vi "Begin.vi"(8 "error in (no error)":errorcluster, 11 "Grabber in":refnum<class "Grabber.lvclass">) -> (0 "error out":errorcluster, 3 "Grabber out":refnum<class "Grabber.lvclass">)   [LabVIEW 2013, in "Grabber.lvclass"]
uses:
  Grabber.lvclass
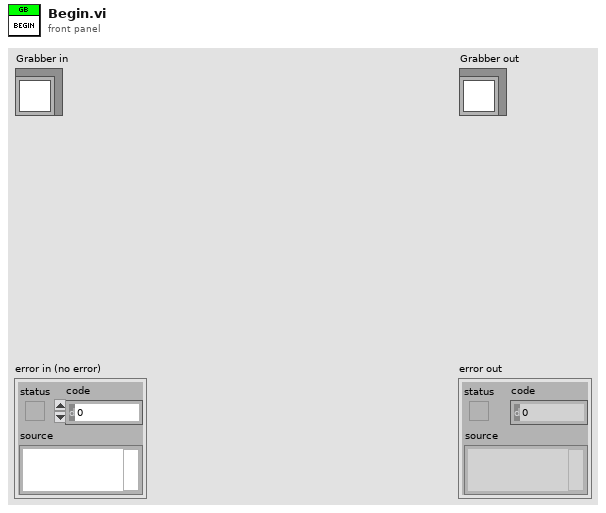
[diagram p1: front panel]
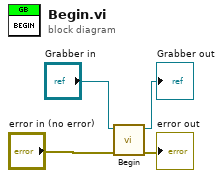
[diagram p0: block diagram]
diagram:
  n1 = call-dynamic "Begin.vi"("error in (no error)"="error in (no error)", "Grabber in"="Grabber in") -> ("error out"=→"error out":errorcluster, "Grabber out"=→"Grabber out":refnum<class "Grabber.lvclass">)  [unwired: 8 in]
